vi "Get number of timers.vi"(8 "error in (no error)":errorcluster) -> (0 "error out":errorcluster, 2 "Timers":string[](array[string]), 3 "Number of timers":i32)   [LabVIEW 2021, in "Named Timers.lvlib"]
uses:
  Named Timers.lvlib
  Timer global variable.vi
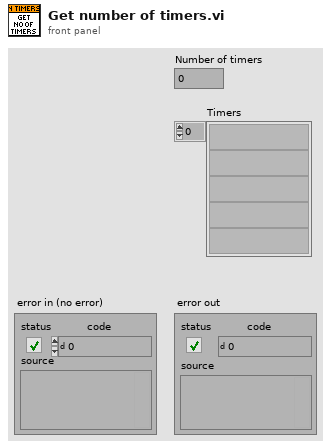
[diagram p1: front panel]
types:
  T1 = typedef "Named Timers.lvlib/Timer Cluster.ctl" = cluster{"Name":string, "Start time (ms)":u32}
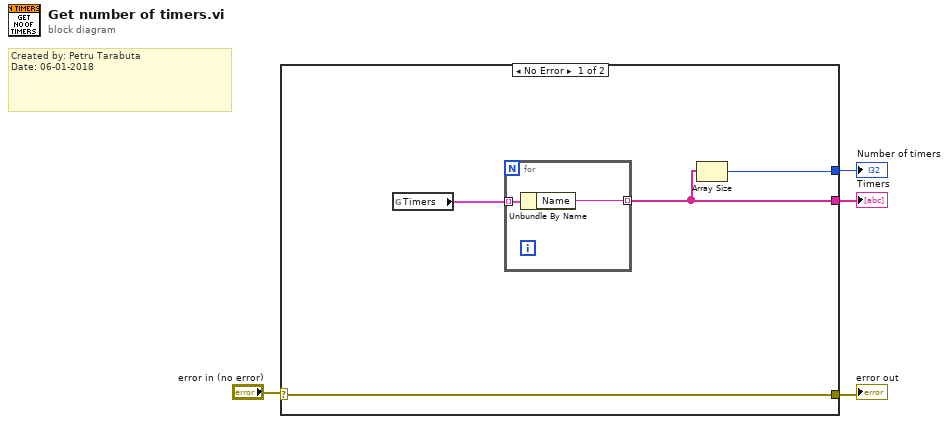
[diagram p0: block diagram]
diagram:
  # "Created by: Petru Tarabuta\nDate: 06-01-2018"
  n1 = case shown="No Error" "error in (no error)" {
    selector: "error in (no error)" -> [w8 w11]
    tunnel: [w8 w11] -> w3
    tunnel: [w6 _] -> w2
    tunnel: [w5 _] -> w1
    frame No Error {
      n2 = global read "Timer global variable.vi" "Timers"() -> (w7:T1[])
      n3 = for {
        tunnel: w7 -> [w10] mode=indexing
        tunnel: [w9] -> w6 mode=indexing
        n4 = Unbundle By Name(w10) -> ("Name"=w9:string)
      }
      n5 = Array Size(array=w6) -> (size(s)=w5:i32)
    }
    frame Error {
    }
  }
  "error out" <- w3
  "Timers" <- w2
  "Number of timers" <- w1
